vi "ApplyOffsetGainToDisplayImage.vi"(6 "Float Image Buffer":T1, 8 "Output mode":enum16{"Corrected Image", "Gain", "Offset"}(ring), 9 "Normalized 1/Gain":sgl[][](array[numeric]), 10 "-Offset":sgl[][](array[numeric]), 11 "Refnum in":T1) -> (2 "Enabled?":bool, 3 "Float Image Buffer":T1)   [LabVIEW 2011]
uses:
  <vilib>/vision/Image Controls.llb/IMAQ Image.ctl
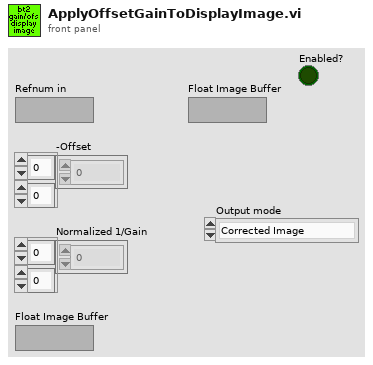
[diagram p1: front panel]
types:
  T1 = typedef "IMAQ Image.ctl" = refnum<image>
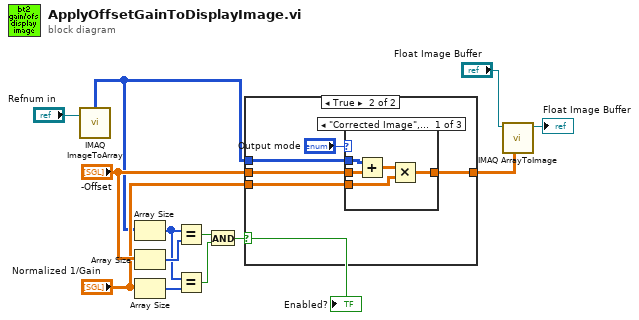
[diagram p0: block diagram]
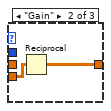
[diagram p3: hidden frame]
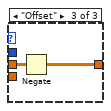
[diagram p4: hidden frame]
diagram:
  n1 = call "IMAQ ImageToArray"("Image"="Refnum in") -> ("Image Pixels (U8)"=w7:u8[][])  [unwired: 3 in, 4 out]
  n2 = Array Size(array=w7) -> (size(s)=w4:i32[])
  n3 = Array Size(array="-Offset") -> (size(s)=w6:i32[])
  n4 = Array Size(array="Normalized 1/Gain") -> (size(s)=w5:i32[])
  n5 = Equal?(x=w4, y=w6) -> (x = y?=w3:bool)
  n6 = Equal?(x=w4, y=w5) -> (x = y?=w2:bool)
  n7 = And(x=w3, y=w2) -> (x .and. y?=w1:bool)
  "Enabled?" <- w1
  n8 = case shown="True" w1 {
    tunnel: [w14 w15] -> w13
    tunnel: "-Offset" -> [_ w17]
    tunnel: "Normalized 1/Gain" -> [_ w16]
    tunnel: w7 -> [w14 w18]
    frame False {
    }
    frame True {
      n9 = case shown="\"Corrected Image\", Default" "Output mode" {
        tunnel: w18 -> [w23 _ _]
        tunnel: w17 -> [w22 _ w28]
        tunnel: w16 -> [w21 w26 _]
        tunnel: [w20 w25 w27] -> w15
        frame "Corrected Image", Default {
          n10 = Add(x=w23, y=w22) -> (x+y=w24:sgl[][])
          n11 = Multiply(x=w24, y=w21) -> (x*y=w20:sgl[][])
        }
        frame "Gain" {
          n12 = Reciprocal(x=w26) -> (1/x=w25:sgl[][])
        }
        frame "Offset" {
          n13 = Negate(x=w28) -> (-x=w27:sgl[][])
        }
      }
    }
  }
  n14 = call "IMAQ ArrayToImage"("Image Pixels (Float)"=w13, "Image"="Float Image Buffer") -> ("Image Out"=→"Float Image Buffer":T1)  [unwired: 8 in, 1 out]
